vi "Green Board Report Voltage Readings.vi"(6 "Message IN":string, 7 "Green Board Enum":T1, 8 "error in (no error)":errorcluster) -> (0 "error out":errorcluster, 1 "Message Out":string, 2 "VISA resource name out":refnum<visa-resource-name>, 5 "Result":dbl)   [LabVIEW 2022 SP3]
uses:
  Serial Board Com/ADCSelector GB.ctl
  <vilib>/Instr/_visa.llb/VISA Flush IO Buffer Mask.ctl
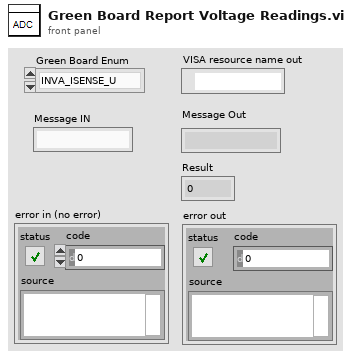
[diagram p1: front panel]
types:
  T1 = typedef "ADCSelector GB.ctl" = enum16{"INVA_ISENSE_U", "INVA_ISENSE_V", "INVA_ISENSE_W", "INVA_UDC", "INVA_TEMP", "HB_ISENSE", "AUX_ISENSE_U", "AUX_ISENSE_V", "AUX_ISENSE_W", "VLINE_AB", "VLINE_BC", "VLINE_CA", "REF_1P5V", "VSENSE_POS_24V", "VSENSE_POS_5V", "VSENSE_NEG_15V", "TEST_POINT", "INVB_ISENSE_U", "INVB_ISENSE_V", "INVB_ISENSE_W", "INVB_UDC", "INVB_TEMP", "HB_TEMP", "AUXA_TEMP", "AUXB_TEMP", "AUXC_TEMP", "VOUT_AB", "VOUT_BC", "VOUT_CA", "REF_2P5V", "VSENSE_POS_15V", "VSENSE_POS_3P3V", "NET_ANALYZER"}
  T2 = typedef "VISA Flush IO Buffer Mask.ctl" = u16
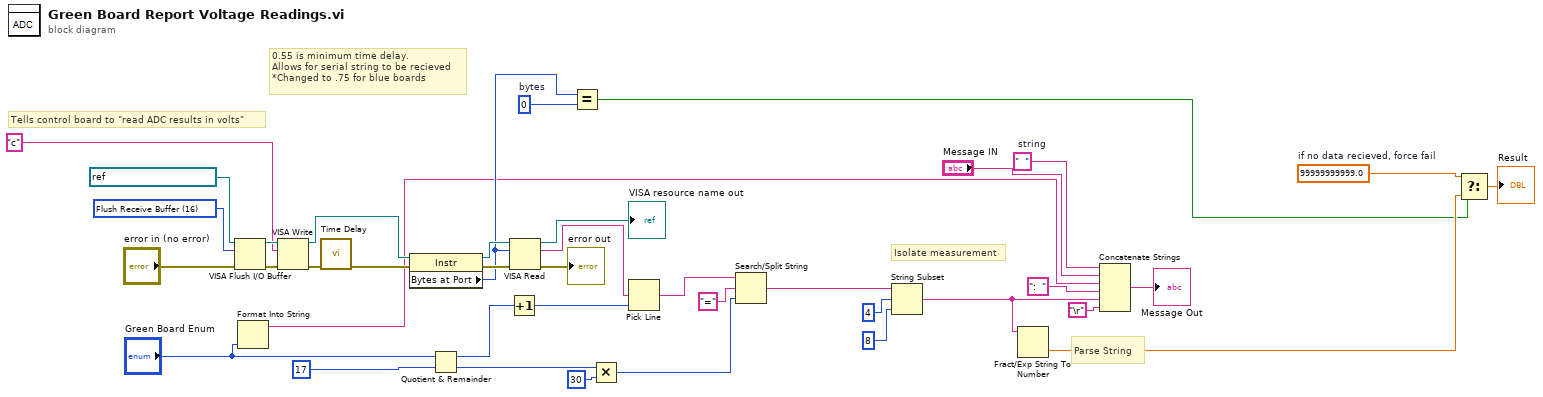
[diagram p0: block diagram]
diagram:
  w10 = "  "  # string
  w15 = 99999999999.0  # if no data recieved, force fail
  w18 = u32 0  # bytes
  w23 = T2 16 items=["Flush Receive Buffer"=16, "Write Transmit Buffer to Device"=32, "Flush Receive Buffer (No I/O)"=64, "Flush Transmit Buffer"=128] ("Mask")
  # "Isolate measurement"
  # "Parse String"
  # "0.55 is minimum time delay.\nAllows for serial string to be recieved\n*Changed to .75 for blue boards"
  # "Tells control board to \"read ADC results in volts\""
  n1 = VISA Flush I/O Buffer(VISA resource name=refnum<visa-resource-name> "ControlBoard", mask (16)=w23, error in (no error)="error in (no error)") -> (VISA resource name out=w25:refnum<visa-resource-name>, error out=w26:errorcluster)
  n2 = Format Into String("Green Board Enum") -> (resulting string=w3:string)  [unwired: 3 in, 1 out]
  n3 = VISA Write(VISA resource name=w25, write buffer="c", error in (no error)=w26) -> (VISA resource name out=w28:refnum<visa-resource-name>, error out=w24:errorcluster)  [unwired: 1 out]
  n4 = call "Time Delay"("error in (no error)"=w24) -> ("error out"=w27:errorcluster)  [unwired: 10 in]
  n5 = property class="Instr"(reference=w28, error in=w27) -> (reference out=w21:refnum<visa-resource-name>, error out=w22:errorcluster, "Bytes at Port"=w19:u32)
  n6 = Quotient & Remainder(x="Green Board Enum", y=17) -> (x-y*floor(x/y)=w32:i32, floor(x/y)=w34:i32)
  n7 = Increment(x=w32) -> (x+1=w33:i32)
  n8 = VISA Read(VISA resource name=w21, byte count=w19, error in (no error)=w22) -> (VISA resource name out=→"VISA resource name out":refnum<visa-resource-name>, read buffer=w37:string, error out=→"error out":errorcluster)  [unwired: 1 out]
  n9 = Equal?(x=w19, y=w18) -> (x = y?=w16:bool)
  n10 = Multiply(x=w34, y=30) -> (x*y=w36:i32)
  n11 = Pick Line(multi-line string=w37, line index=w33) -> (output string=w38:string)  [unwired: 1 in]
  n12 = Search/Split String(string=w38, search string/char (-)="=" ("regular expression"), offset (0)=w36) -> (match + rest of string=w30:string)  [unwired: 2 out]
  n13 = String Subset(string=w30, offset (0)=4, length (rest)=8 ("offset (0)")) -> (substring=w12:string)
  n14 = Fract/Exp String To Number(string=w12) -> (number=w17:dbl)  [unwired: 3 in, 1 out]
  n15 = Concatenate Strings(w10, "Message IN", w3, ":  ", w12, "\r") -> (→"Message Out":string)
  n16 = Select(t=w15, s=w16, f=w17) -> (s? t:f=→"Result":dbl)
